vi "Get SLSC Lib Version.vi"(8 "error in (no error)":errorcluster, 11 "bitfile path":path) -> (0 "error out":errorcluster, 1 "valid bitfile":bool, 2 "SLSC version enum":T1, 3 "vi info":T2 {"RegisterMap"."Address" format="%.0x"}, 5 "SLSC version string":string)   [LabVIEW 2014, in "SLSC configuration System Explorer.lvlib"]
uses:
  SLSC configuration System Explorer.lvlib
  <vilib>/rvi/Bitfile/niFpgaBitfileStructure_VI.ctl
  <vilib>/rvi/Bitfile/nirviControlStructure.ctl
  <vilib>/rvi/Bitfile/nirviTypdefDescription.ctl
  <vilib>/rvi/Bitfile/nirviMechanicalAction.ctl
  <vilib>/rvi/Bitfile/nirviSubControlStructure.ctl
  <vilib>/rvi/Bitfile/nirviClusterElementControl.ctl
  <vilib>/picture/picture.llb/imagedata.ctl
  Type Defs/SLSC Custom Device Version.ctl
  <vilib>/Utility/VariantDataType/VariantType.lvlib
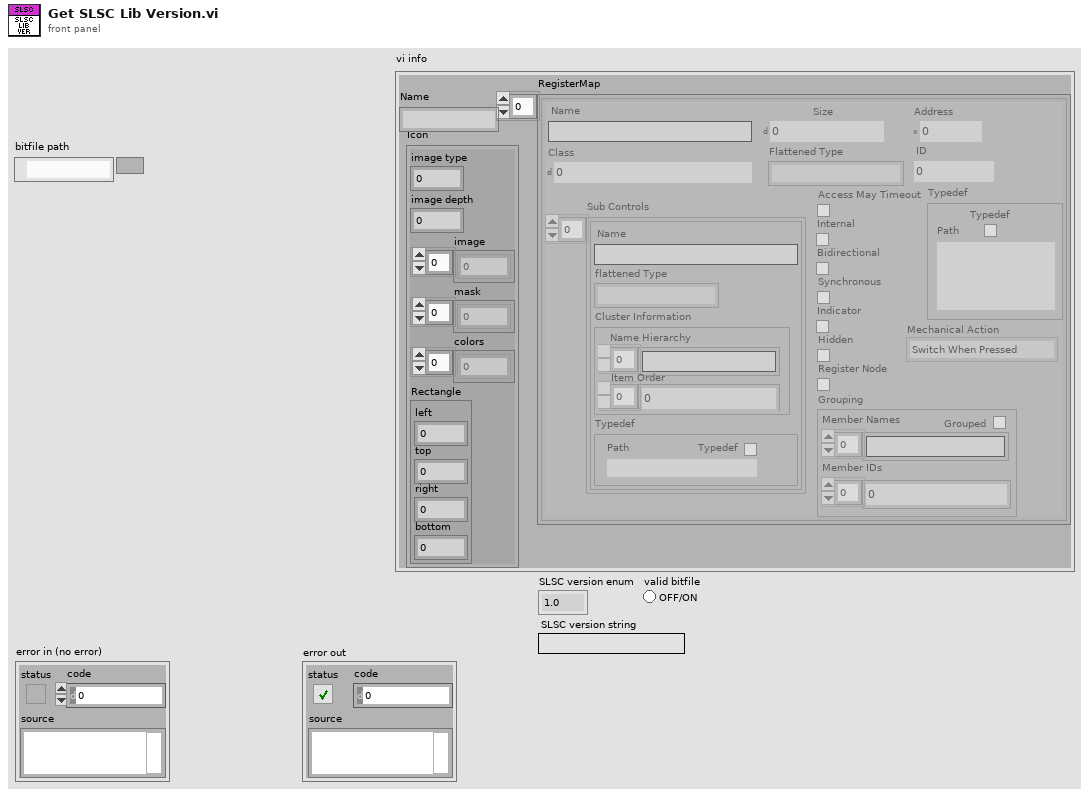
[diagram p1: front panel]
types:
  T1 = typedef "SLSC configuration System Explorer.lvlib/SLSC Custom Device Version.ctl" = enum8{"1.0"}
  T2 = typedef "niFpgaBitfileStructure_VI.ctl" = cluster{"Name":string, "RegisterMap":T3[], "Icon":T8}
  T3 = typedef "nirviControlStructure.ctl" = cluster{"Name":string, "Hidden":bool, "Indicator":bool, "Flattened Type":string, "Grouping":cluster{"Grouped":bool, "Member Names":string[], "Member IDs":u32[]}, "Address":u32, "Size":u32, "Class":u32, "Internal":bool, "Typedef":T4, "ID":u32, "Bidirectional":bool, "Synchronous":bool, "Mechanical Action":T5, "Sub Controls":T6[], "Access May Timeout":bool, "Register Node":bool}
  T4 = typedef "nirviTypdefDescription.ctl" = cluster{"Typedef":bool, "Path":path}
  T5 = typedef "nirviMechanicalAction.ctl" = enum8{"Switch When Pressed", "Switch When Released", "Switch Until Released", "Latch When Pressed", "Latch When Released", "Latch Until Released"}
  T6 = typedef "nirviSubControlStructure.ctl" = cluster{"Name":string, "flattened Type":string, "Cluster Information":T7, "Typedef":T4}
  T7 = typedef "nirviClusterElementControl.ctl" = cluster{"Name Hierarchy":string[], "Item Order":u32[]}
  T8 = typedef "imagedata.ctl" = cluster{"image type":i32, "image depth":i32, "image":u8[], "mask":u8[], "colors":u32[], "Rectangle":cluster{"left":i16, "top":i16, "right":i16, "bottom":i16}}
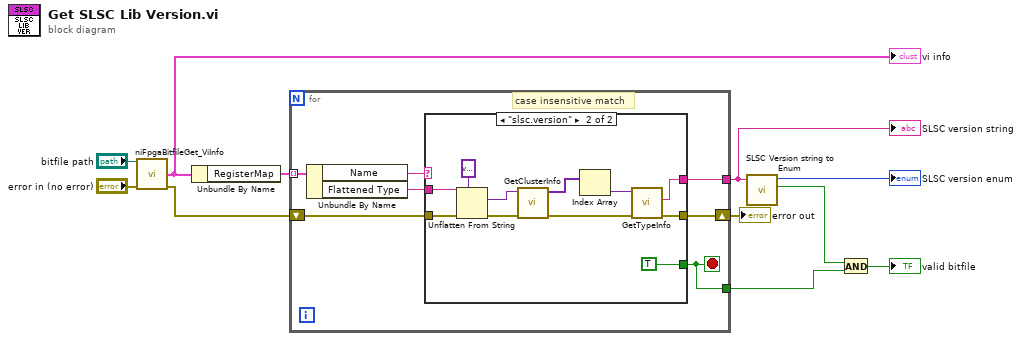
[diagram p0: block diagram]
diagram:
  n1 = call <vilib>:"niFpgaBitfileGet_ViInfo.vi"("bitfile path"="bitfile path", "error in (no error)"="error in (no error)") -> ("vi info"=w8:T2, "error out"=w7:errorcluster)  [unwired: 1 in, 11 out]
  "vi info" <- w8
  n2 = Unbundle By Name(w8) -> ("RegisterMap"=w9:T3[])
  n3 = for {
    shift-right: [w14] -> w2
    shift-left: w7 -> [w18]
    tunnel: w9 -> [w17] mode=indexing
    tunnel: [w13] -> w4
    tunnel: [w12] -> w6
    stop <- w13 stop-if-true
    # "case insensitive match"
    n4 = Unbundle By Name(w17) -> ("Name"=w16:string, "Flattened Type"=w15:string)
    n5 = case shown="\"slsc.version\"" w16 {
      tunnel: w18 -> [w19 w25]
      tunnel: w15 -> [_ w24]
      tunnel: [w19 w27] -> w14
      tunnel: [_ TRUE] -> w13
      tunnel: [_ w20] -> w12
      frame Default {
      }
      frame "slsc.version" {
        n6 = Unflatten From String(type=variant ("Variant"), binary string=w24, error in (no error)=w25) -> (value=w22:variant, error out=w23:errorcluster)  [unwired: 3 out]
        n7 = call <vilib>:"GetClusterInfo.vi"("error in (no error)"=w23, "Variant"=w22) -> ("error out"=w29:errorcluster, "Cluster Elements"=w30:variant[])  [unwired: 8 in]
        n8 = Index Array(array=w30) -> (element=w28:variant)  [unwired: 1 in]
        n9 = call <vilib>:"GetTypeInfo.vi"("error in (no error)"=w29, "Variant"=w28) -> ("error out"=w27:errorcluster, "Name"=w20:string)  [unwired: 5 in, 3 out]
      }
    }
  }
  "error out" <- w2
  "SLSC version string" <- w6
  n10 = call "SLSC Version string to Enum.vi"("SLSC version string"=w6) -> ("valid"=w5:bool, "SLSC version enum"=→"SLSC version enum":T1)  [unwired: 9 in]
  n11 = And(x=w5, y=w4) -> (x .and. y?=→"valid bitfile":bool)
